vi "close references.vi"(0 "Watchdog":refnum<queue>, 1 "Calibration":refnum<queue>, 5 "Processing":refnum<queue>, 7 "Acquisition":refnum<queue>, 9 "RFID":refnum<queue>, 11 "error in (no error)":errorcluster) -> (15 "error out":errorcluster)   [LabVIEW 2015]
uses:
  Message Queue/Message Cluster.ctl
  Message Queue/Enqueue Message (Single).vi
  Message Queue/Message Queue.lvlib
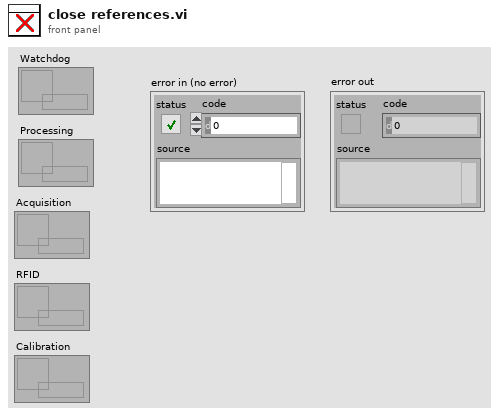
[diagram p1: front panel]
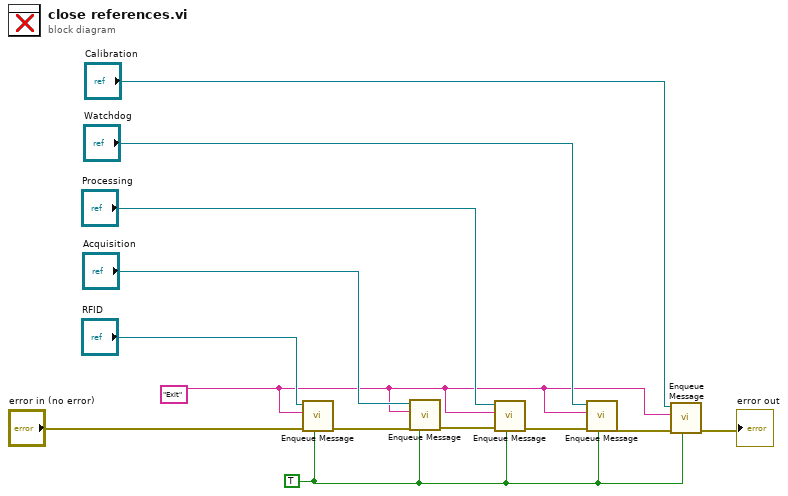
[diagram p0: block diagram]
diagram:
  w1 = TRUE ("Priority Message? (F)")
  w2 = "Exit" ("Message")
  n1 = call-poly "Enqueue Message.vi"("Priority Message? (F)"=w1, "error in (no error)"="error in (no error)", "Message"=w2, "Message Queue"="RFID") -> ("error out"=w12:errorcluster)  [unwired: 6 in, 1 out]
  n2 = call-poly "Enqueue Message.vi"("Priority Message? (F)"=w1, "error in (no error)"=w12, "Message"=w2, "Message Queue"="Acquisition") -> ("error out"=w7:errorcluster)  [unwired: 6 in, 1 out]
  n3 = call-poly "Enqueue Message.vi"("Priority Message? (F)"=w1, "error in (no error)"=w7, "Message"=w2, "Message Queue"="Processing") -> ("error out"=w6:errorcluster)  [unwired: 6 in, 1 out]
  n4 = call-poly "Enqueue Message.vi"("Priority Message? (F)"=w1, "error in (no error)"=w6, "Message"=w2, "Message Queue"="Watchdog") -> ("error out"=w5:errorcluster)  [unwired: 6 in, 1 out]
  n5 = call-poly "Enqueue Message.vi"("Priority Message? (F)"=w1, "error in (no error)"=w5, "Message"=w2, "Message Queue"="Calibration") -> ("error out"=→"error out":errorcluster)  [unwired: 6 in, 1 out]
